vi "Switch Map Scan List.vi"(8 "error in (no error)":errorcluster, 10 "JSONCluster":T1, 11 "Ch Spreadsheet":path=path "/home/lvuser/Chad_Test.csv") -> (0 "error out":errorcluster, 2 "IVI Specifications":string[][](array[string]), 3 "Channel Specs":string[][](array[string]))   [LabVIEW 2019]
uses:
  JSONCluster.ctl
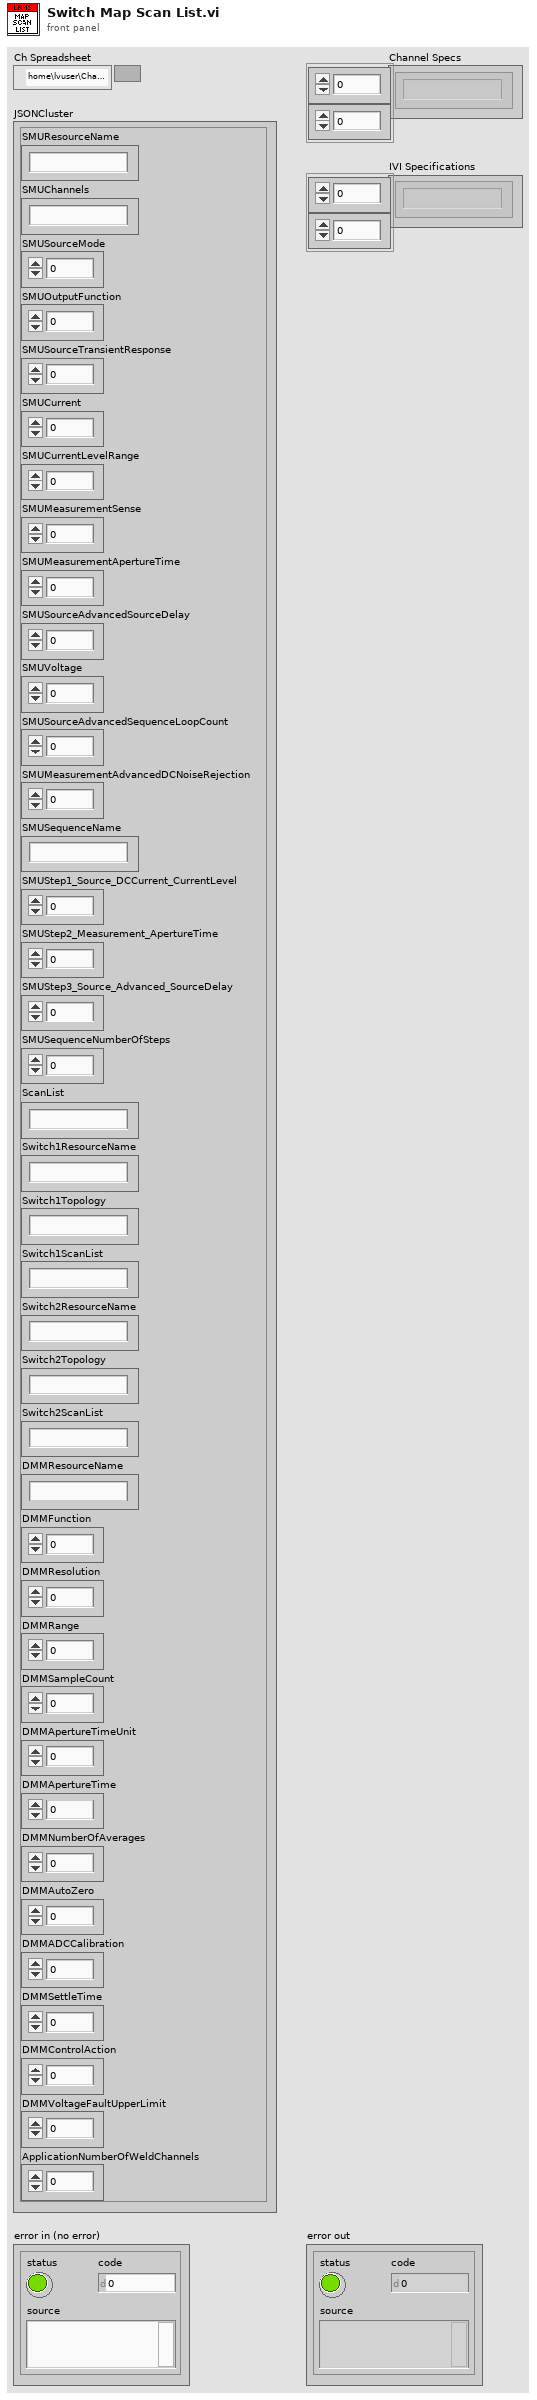
[diagram p1: front panel]
types:
  T1 = typedef "JSONCluster.ctl" = cluster{"SMUResourceName":string, "SMUChannels":string, "SMUSourceMode":i32, "SMUOutputFunction":i32, "SMUSourceTransientResponse":i32, "SMUCurrent":dbl, "SMUCurrentLevelRange":dbl, "SMUMeasurementSense":i32, "SMUMeasurementApertureTime":dbl, "SMUSourceAdvancedSourceDelay":dbl, "SMUVoltage":dbl, "SMUSourceAdvancedSequenceLoopCount":i32, "SMUMeasurementAdvancedDCNoiseRejection":i32, "SMUSequenceName":string, "SMUStep1_Source_DCCurrent_CurrentLevel":i32, "SMUStep2_Measurement_ApertureTime":i32, "SMUStep3_Source_Advanced_SourceDelay":i32, "SMUSequenceNumberOfSteps":i32, "ScanList":string, "Switch1ResourceName":string, "Switch1Topology":string, "Switch1ScanList":string, "Switch2ResourceName":string, "Switch2Topology":string, "Switch2ScanList":string, "DMMResourceName":string, "DMMFunction":i32, "DMMResolution":dbl, "DMMRange":dbl, "DMMSampleCount":i32, "DMMApertureTimeUnit":i32, "DMMApertureTime":dbl, "DMMNumberOfAverages":i32, "DMMAutoZero":i32, "DMMADCCalibration":i32, "DMMSettleTime":dbl, "DMMControlAction":i32, "DMMVoltageFaultUpperLimit":dbl, "ApplicationNumberOfWeldChannels":i32}
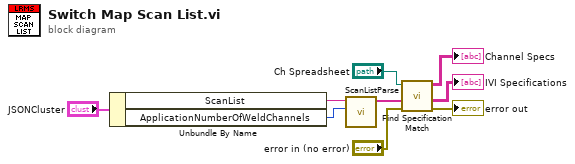
[diagram p0: block diagram]
diagram:
  n1 = Unbundle By Name("JSONCluster") -> ("ScanList"=w5:string, "ApplicationNumberOfWeldChannels"=w6:i32)
  n2 = call "ScanListParse.vi"("ApplicationNumberOfWeldChannels"=w6, "Input"=w5) -> ("Output"=w8:string[])  [unwired: 9 in]
  n3 = call "Find Specification Match.vi"("error in (no error)"="error in (no error)", "Channel List"=w8, "file path (dialog if empty)"="Ch Spreadsheet") -> ("error out"=→"error out":errorcluster, "IVI Specifications"=→"IVI Specifications":string[][], "Channel Specs"=→"Channel Specs":string[][])  [unwired: 5 in]
